vi "SMOVE.vi"(0 "refnum in":refnum<vi>, 5 "Source":string, 7 "Destination":string, 9 "Member":string, 11 "error in":errorcluster) -> (4 "refnum out":refnum<vi>, 6 "Data":T1, 15 "error out":errorcluster)   [LabVIEW 2020]
uses:
  SubVIs/Controls/redis-data.ctl
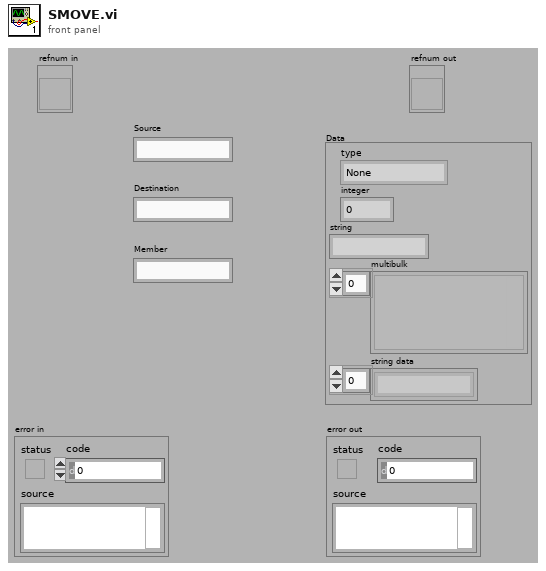
[diagram p1: front panel]
types:
  T1 = typedef "redis-data.ctl" = cluster{"type":enum16{"None", "Error", "Status", "Nil", "Integer", "String", "Multibulk"}, "integer":i64, "string":string, "multibulk":variant[], "string data":string[]}
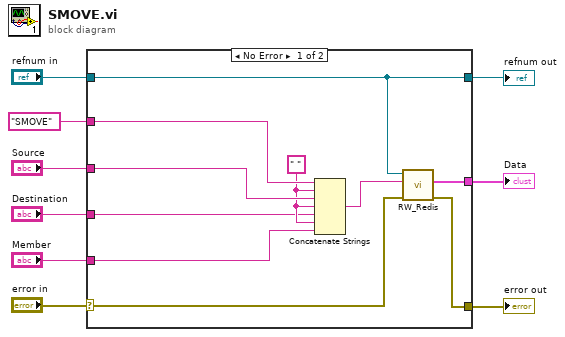
[diagram p0: block diagram]
diagram:
  n1 = case shown="No Error" "error in" {
    selector: "error in" -> [w17 w21]
    tunnel: "SMOVE" -> [w19 _]
    tunnel: "refnum in" -> [w14 w20]
    tunnel: [w16 w21] -> w6
    tunnel: [w15 _] -> w5
    tunnel: [w14 w20] -> w4
    tunnel: "Member" -> [w10 _]
    tunnel: "Destination" -> [w11 _]
    tunnel: "Source" -> [w13 _]
    frame No Error {
      w12 = " "
      n2 = Concatenate Strings(w19, w12, w13, w12, w11, w12, w10) -> (w18:string)
      n3 = call "RW_Redis.vi"("error in"=w17, "command"=w18, "refnum"=w14) -> ("error out"=w16:errorcluster, "Data"=w15:T1)  [unwired: 7 in]
    }
    frame Error {
    }
  }
  "error out" <- w6
  "Data" <- w5
  "refnum out" <- w4
